vi "Pockels Cal-Write external condit globals.vi"(11 "Pockels Cal table":string[][](array[string])) -> ()   [LabVIEW 2013]
uses:
  Globals/gl_Calibration globals.vi
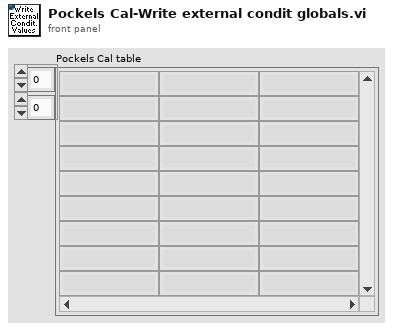
[diagram p1: front panel]
types:
  T1 = typedef "Pockels cal conditions cluster.ctl" = cluster{"Wavelength":u16, "Zoom":u8, "Dwell time (us)":dbl, "Pockels bias":i16, "Prism 1":u16, "Prism 2":u16, "Laser power during pockels cal (mW)":u16}
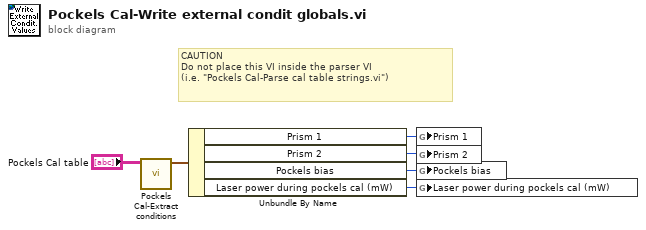
[diagram p0: block diagram]
diagram:
  # "CAUTION\nDo not place this VI inside the parser VI \n(i.e. \"Pockels Cal-Parse cal table strings.vi\")"
  n1 = call "Pockels Cal-Extract conditions.vi"("Pockels Cal table (full)"="Pockels Cal table") -> ("Pockels cal conditions"=w2:T1)  [unwired: 8 in, 2 out]
  n2 = Unbundle By Name(w2) -> ("Prism 1"=w5:u16, "Prism 2"=w4:u16, "Pockels bias"=w3:i16, "Laser power during pockels cal (mW)"=w1:u16)
  n3 = global write "gl_Calibration globals.vi" "Prism 1"(w5) -> ()
  n4 = global write "gl_Calibration globals.vi" "Prism 2"(w4) -> ()
  n5 = global write "gl_Calibration globals.vi" "Pockels bias"(w3) -> ()
  n6 = global write "gl_Calibration globals.vi" "Laser power during pockels cal (mW)"(w1) -> ()
